vi "Shutdown Window.vi"(8 "error in (no error)":errorcluster, 11 "Window":T1) -> (0 "error out":errorcluster)   [LabVIEW 2015, in "Main Controller Actor API.lvclass"]
uses:
  Main Controller Actor API.lvclass
  Actor/Windows.ctl
  Re-use Libraries/Minimal Actor Framework/Messaging/Message/Message.lvclass/Message.ctl
  Globals.vi
  Re-use Libraries/Minimal Actor Framework/Messaging/Message/Message.lvclass
  Actor/Main Controller Actor.lvclass
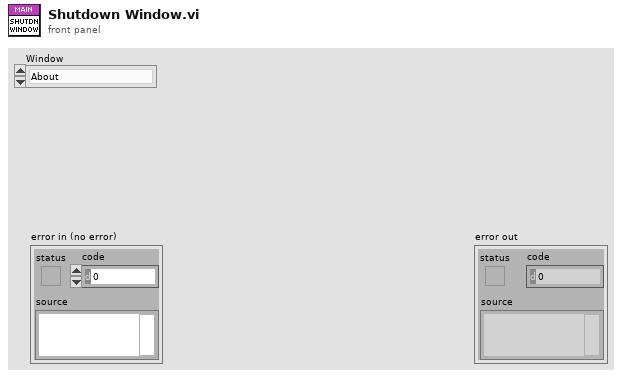
[diagram p1: front panel]
types:
  T1 = typedef "Main Controller Actor.lvclass/Windows.ctl" = enum16{"About", "Status", "Debugger"}
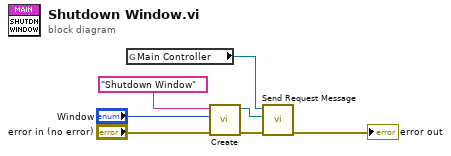
[diagram p0: block diagram]
diagram:
  n1 = global read "Globals.vi" "Main Controller"() -> (w3:refnum<class "Main Controller Actor API.lvclass">)
  n2 = call "Create.vi"("error in (no error)"="error in (no error)", "Data"="Window", "Name"="Shutdown Window" ("Parameter")) -> ("error out"=w4:errorcluster, "Message out"=w5:refnum<class "Message.lvclass">)  [unwired: 7 in]
  n3 = call-dynamic "Send Request Message.vi"("error in (no error)"=w4, "Message"=w5, "Actor API in"=w3) -> ("error out"=→"error out":errorcluster)  [unwired: 8 in]
